vi "List Acquire.vi"(8 "error in (no error)":errorcluster, 9 "List Notifier":refnum<notifier>, 10 "Data Queue":refnum<queue>, 11 "Hardware Resources in":T2 {"Baud Rate" items=["<0>"=0, "4800"=4800, "9600"=9600, "19200"=19200, "38400"=38400, "57600"=57600, "115200"=115200]}) -> (0 "error out":errorcluster, 3 "Hardware Resources out":T2 {"Baud Rate" items=["<0>"=0, "4800"=4800, "9600"=9600, "19200"=19200, "38400"=38400, "57600"=57600, "115200"=115200]})   [LabVIEW 2022 SP3, in "Acquisition.lvlib"]
doc: "Perform the acquisition. Replace the contents of this diagram with calls to acquisition hardware."
uses:
  Acquisition.lvlib
  Hardware Configuration.ctl
  <instrlib>/BK Precision 911X Series/BK Precision 911X Series.lvlib
panel:
  in  "Meas Out":T1
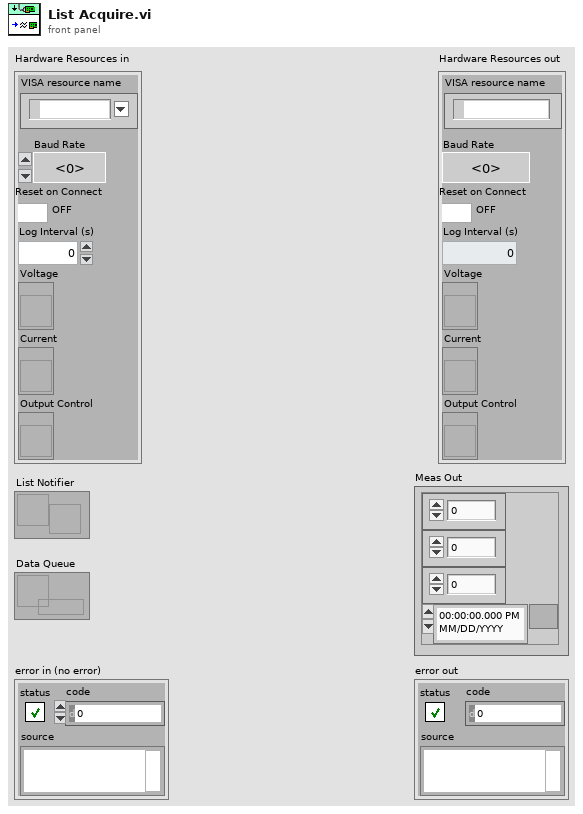
[diagram p1: front panel]
types:
  T1 = cluster{"Voltage":dbl, "Current":dbl, "Power":dbl, timestamp}
  T2 = typedef "Acquisition.lvlib/Hardware Configuration.ctl" = cluster{"VISA resource name":refnum<visa-resource-name>, "Baud Rate":u32, "Reset on Connect":bool, "Log Interval (s)":dbl, "Voltage":refnum<vi>, "Current":refnum<vi>, "Output Control":refnum<vi>}
  T3 = cluster{"List Stop COND":i32, "Voltage":dbl, "Current":dbl, "Power":dbl}
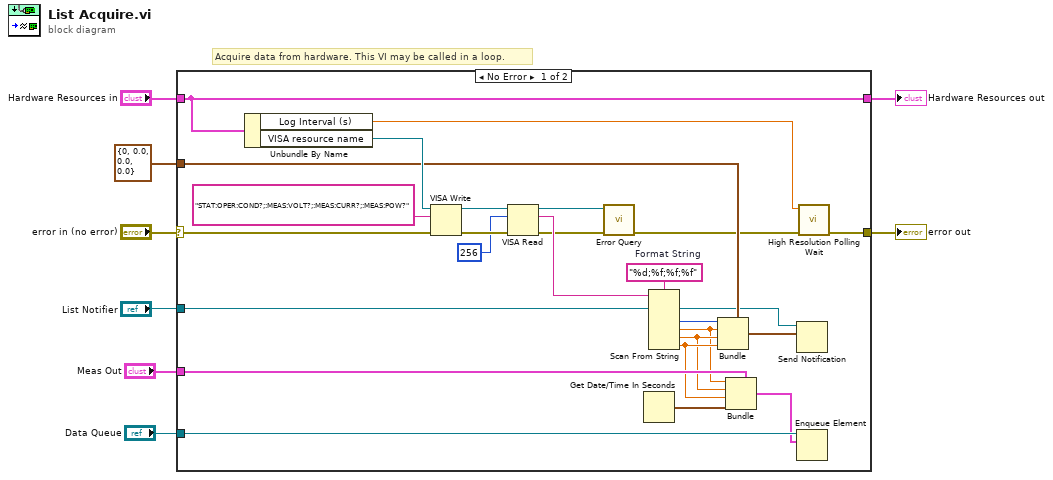
[diagram p0: block diagram]
diagram:
  # "Acquire data from hardware. This VI may be called in a loop."
  n1 = case shown="No Error" "error in (no error)" {
    selector: "error in (no error)" -> [w30 w34]
    tunnel: [w22 w34] -> w7
    tunnel: "Hardware Resources in" -> [w33 w35]
    tunnel: [w33 w35] -> w5
    tunnel: T3 {"List Stop COND"=0, "Voltage"=0.0, "Current"=0.0, "Power"=0.0} ("List Data Out") -> [w25 _]
    tunnel: "List Notifier" -> [w24 _]
    tunnel: "Data Queue" -> [w17 _]
    tunnel: "Meas Out" -> [w15 _]
    frame No Error {
      w27 = "%d;%f;%f;%f"  # Format String
      n2 = Unbundle By Name(w33) -> ("Log Interval (s)"=w9:dbl, "VISA resource name"=w31:refnum<visa-resource-name>)
      n3 = VISA Write(VISA resource name=w31, write buffer="STAT:OPER:COND?;:MEAS:VOLT?;:MEAS:CURR?;:MEAS:POW?", error in (no error)=w30) -> (VISA resource name out=w29:refnum<visa-resource-name>, error out=w28:errorcluster)  [unwired: 1 out]
      n4 = VISA Read(VISA resource name=w29, byte count=u32 256, error in (no error)=w28) -> (VISA resource name out=w19:refnum<visa-resource-name>, read buffer=w26:string, error out=w21:errorcluster)  [unwired: 1 out]
      n5 = call <instrlib>:"Error Query.vi"("error in (no error)"=w21, "VISA resource name"=w19) -> ("error out"=w20:errorcluster)  [unwired: 6 in, 3 out]
      n6 = Get Date/Time In Seconds() -> (seconds since 1Jan1904=w13:timestamp)
      n7 = Scan From String(format string=w27, input string=w26) -> (output 1=w18:i32, output 2=w10:dbl, output 3=w11:dbl, output 4=w12:dbl)  [unwired: 6 in, 3 out]
      n8 = Bundle(cluster=w25, "List Stop COND"=w18, "Voltage"=w10, "Current"=w11, "Power"=w12) -> (w16:T3)
      n9 = Bundle(cluster=w15, "Voltage"=w10, "Current"=w11, "Power"=w12, w13) -> (w14:T1)
      n10 = Send Notification(notification=w16, notifier=w24) -> ()  [unwired: 1 in, 2 out]
      n11 = Enqueue Element(queue=w17, element=w14) -> ()  [unwired: 2 in, 3 out]
      n12 = call <vilib>:"High Resolution Polling Wait.vi"("error in (no error)"=w20, "seconds to wait"=w9) -> ("error out"=w22:errorcluster)  [unwired: 9 in]
    }
    frame Error {
    }
  }
  "Hardware Resources out" <- w5
  "error out" <- w7
